vi "Read transformedData.vi"(8 "error in (no error)":errorcluster, 11 "SoundAO.lvclass in":refnum<class "SoundAO.lvclass">) -> (0 "error out":errorcluster, 2 "transformedData":dbl[][](array[numeric]), 3 "SoundAO.lvclass out":refnum<class "SoundAO.lvclass">)   [LabVIEW 2009, in "Hardware.lvlib" / "Channels.lvlib" / "SoundAO.lvclass"]
uses:
  SoundAO.lvclass
  SoundAO.lvclass/SoundAO.ctl
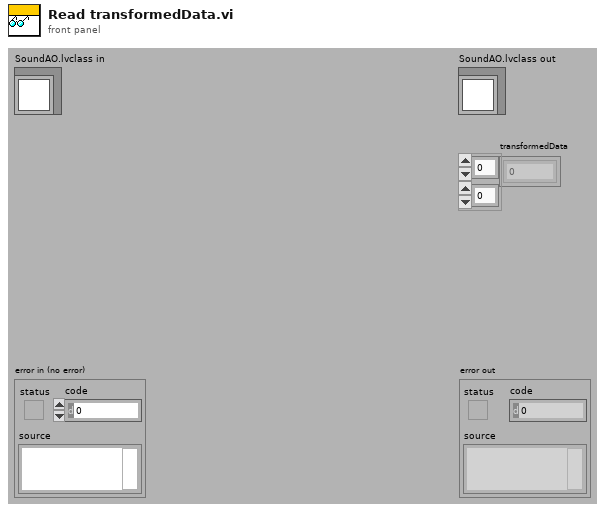
[diagram p1: front panel]
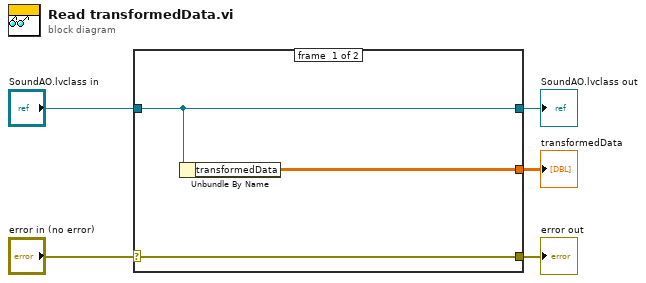
[diagram p0: block diagram]
diagram:
  n1 = case shown="No Error" "error in (no error)" {
    selector: "error in (no error)" -> [w8 w9]
    tunnel: [w8 w9] -> w4
    tunnel: [w7 w10] -> w2
    tunnel: "SoundAO.lvclass in" -> [w7 w10]
    tunnel: [w6 _] -> w1
    frame #0 {
      n2 = Unbundle By Name(w7) -> ("transformedData"=w6:dbl[][])
    }
    frame #1 {
    }
  }
  "error out" <- w4
  "SoundAO.lvclass out" <- w2
  "transformedData" <- w1
